vi "wrap.vi"(7 "Max":i32, 11 "value":i32) -> (2 "wrapped?":bool, 3 "wrapped value":i32)   [LabVIEW 2021, in "d22.lvlib"]
uses:
  d22.lvlib
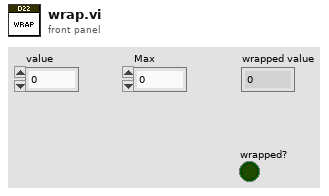
[diagram p1: front panel]
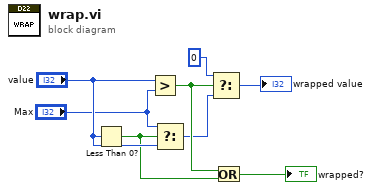
[diagram p0: block diagram]
diagram:
  n1 = Less Than 0?(x="value") -> (x < 0?=w1:bool)
  n2 = Greater?(x="value", y="Max") -> (0:w8:bool)
  n3 = Select(t="Max", s=w1, f="value") -> (s? t:f=w6:i32)
  n4 = Select(t=0, s=w8, f=w6) -> (s? t:f=→"wrapped value":i32)
  n5 = Or(x=w8, y=w1) -> (x .or. y?=→"wrapped?":bool)
